vi "Axis_to_Button.vi"(11 "Axis":dbl) -> (3 "Signal":bool)   [LabVIEW 2014]
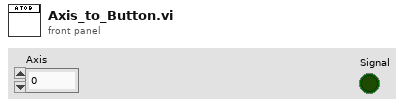
[diagram p1: front panel]
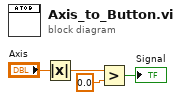
[diagram p0: block diagram]
diagram:
  n1 = Absolute Value(x="Axis") -> (abs(x)=w3:dbl)
  n2 = Greater?(x=w3, y=0.0 ("Axis 2")) -> (0:→"Signal":bool)
